vi "RT Simulation.vi"() -> ()   [LabVIEW 2014]
panel:
  out "error out":errorcluster
  out "String":string
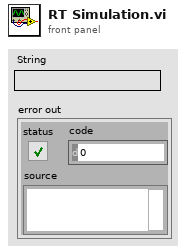
[diagram p1: front panel]
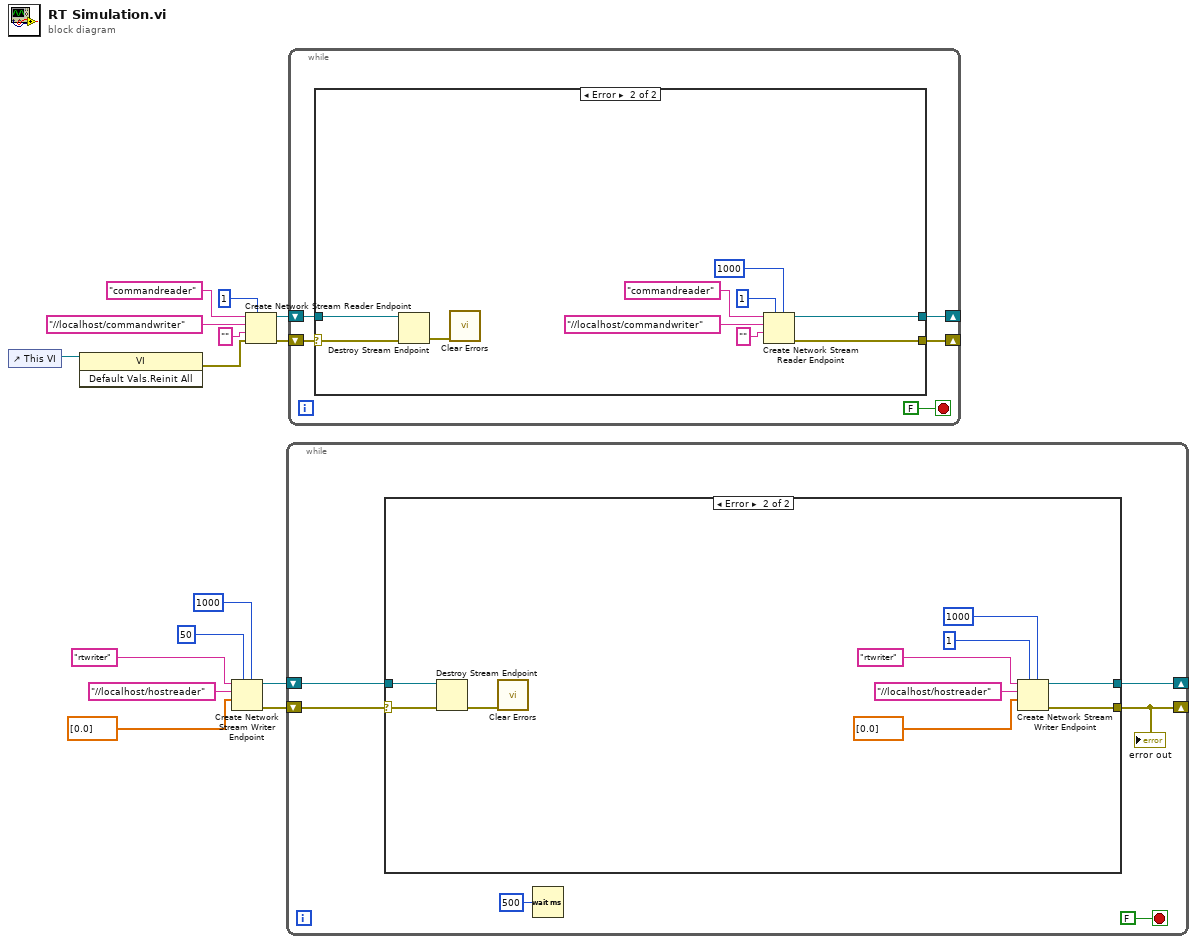
[diagram p0: block diagram]
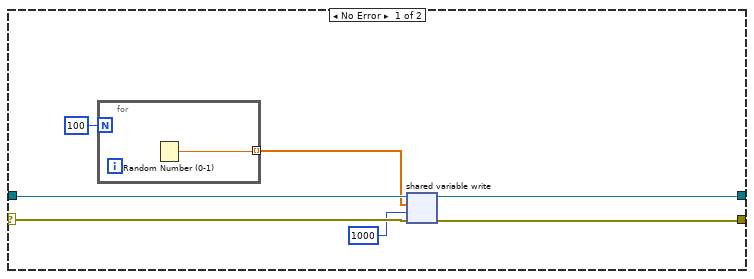
[diagram p2: hidden frame]
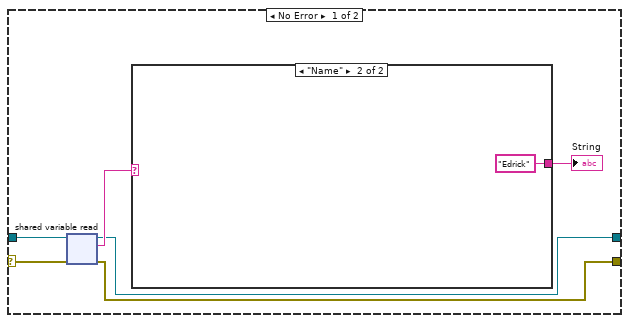
[diagram p3: hidden frame]
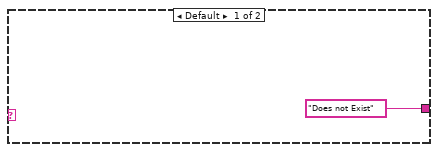
[diagram p4: hidden frame]
diagram:
  n1 = control-ref of="This VI"() -> (w9:refnum<vi>)
  n2 = invoke class="VI" method="Default Vals.Reinit All"(reference=w9) -> (error out=w8:errorcluster)  [unwired: 2 in, 2 out]
  n3 = Create Network Stream Writer Endpoint(5:1000 ("timeout in ms (-1)"), 7:50 ("writer buffer size"), 9:dbl[] [0.0], 10:"//localhost/hostreader" ("reader url"), 11:"rtwriter" ("writer name")) -> (0:w3:errorcluster, 3:w4:refnum<k21>)  [unwired: 2 in]
  n4 = Create Network Stream Reader Endpoint(7:1 ("reader buffer size"), 8:w8, 9:"" ("reader name"), 10:"//localhost/commandwriter" ("writer name"), 11:"commandreader" ("reader name")) -> (0:w11:errorcluster, 3:w10:refnum<k21>)  [unwired: 2 in]
  n5 = while {
    shift-right: [w18] -> _
    shift-left: w4 -> [w19]
    shift-right: [w17] -> _
    shift-left: w3 -> [w20]
    stop <- FALSE stop-if-true
    n6 = case shown="Error" w20 {
      selector: w20 -> [w23 w36]
      tunnel: w19 -> [w28 w35]
      tunnel: [w27 w31] -> w18
      tunnel: [w26 w30] -> w17
      frame No Error {
        n7 = for {
          N: 100 -> [_]
          tunnel: [w29] -> w24 mode=indexing
          n8 = Random Number (0-1)() -> (number: 0 to 1=w29:dbl)
        }
        n9 = shared-variable-write(w28, w23, w24, 1000 ("timeout ms (-1)")) -> (w27:refnum<k21>, w26:errorcluster)  [unwired: 1 out]
      }
      frame Error {
        n10 = Destroy Stream Endpoint(8:w36, 11:w35) -> (0:w34:errorcluster)
        n11 = call <vilib>:"Clear Errors.vi"("error in (no error)"=w34) -> ()  [unwired: 5 in, 2 out]
        n12 = Create Network Stream Writer Endpoint(5:1000 ("timeout in ms (-1)"), 7:1 ("writer buffer size"), 9:dbl[] [0.0], 10:"//localhost/hostreader" ("reader url"), 11:"rtwriter" ("writer name")) -> (0:w30:errorcluster, 3:w31:refnum<k21>)  [unwired: 2 in]
      }
    }
    "error out" <- w17
    n13 = Wait (ms)(milliseconds to wait=u32 500) -> ()  [unwired: 1 out]
  }
  n14 = while {
    shift-right: [w41] -> _
    shift-left: w10 -> [w42]
    shift-right: [w40] -> _
    shift-left: w11 -> [w43]
    stop <- FALSE stop-if-true
    n15 = case shown="Error" w43 {
      selector: w43 -> [w49 w62]
      tunnel: w42 -> [w50 w61]
      tunnel: [w47 w54] -> w41
      tunnel: [w46 w53] -> w40
      frame No Error {
        n16 = shared-variable-read(w50, w49) -> (w47:refnum<k21>, w46:errorcluster, w48:string)  [unwired: 1 in, 1 out]
        n17 = case shown="\"Name\"" w48 {
          tunnel: ["Does not Exist" ("String") "Edrick" ("String")] -> w45
          frame Default {
          }
          frame "Name" {
          }
        }
        "String" <- w45
      }
      frame Error {
        n18 = Destroy Stream Endpoint(8:w62, 11:w61) -> (0:w60:errorcluster)
        n19 = call <vilib>:"Clear Errors.vi"("error in (no error)"=w60) -> ()  [unwired: 5 in, 2 out]
        n20 = Create Network Stream Reader Endpoint(5:1000 ("timeout in ms (-1)"), 7:1 ("reader buffer size"), 9:"" ("reader name"), 10:"//localhost/commandwriter" ("writer name"), 11:"commandreader" ("reader name")) -> (0:w53:errorcluster, 3:w54:refnum<k21>)  [unwired: 2 in]
      }
    }
  }
